vi "Write ready to log boolean.vi"(8 "error in (no error)":errorcluster, 10 "Ready to Log":bool, 11 "Abstract Display in":refnum<class "Abstract Display.lvclass">) -> (0 "error out":errorcluster, 3 "Abstract Display out":refnum<class "Abstract Display.lvclass">)   [LabVIEW 2014, in "Display Panel.lvlib" / "Abstract Display.lvclass"]
uses:
  Abstract Display.lvclass
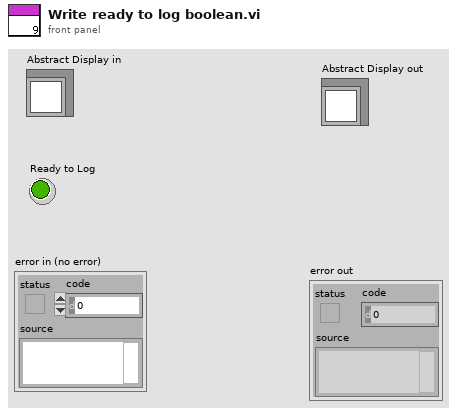
[diagram p1: front panel]
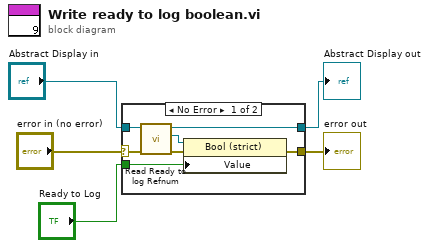
[diagram p0: block diagram]
diagram:
  n1 = case shown="No Error" "error in (no error)" {
    selector: "error in (no error)" -> [w7 w13]
    tunnel: [w12 w13] -> w4
    tunnel: [w10 w14] -> w2
    tunnel: "Abstract Display in" -> [w11 w14]
    tunnel: "Ready to Log" -> [w8 _]
    frame No Error {
      n2 = call-dynamic "Read Ready to log Refnum.vi"("error in (no error)"=w7, "Abstract Display in"=w11) -> ("error out"=w6:errorcluster, "Ready to log Refnum"=w9:refnum<vi>, "Abstract Display out"=w10:refnum<class "Abstract Display.lvclass">)  [unwired: 7 in]
      n3 = property class="Bool (strict)"(reference=w9, error in=w6, "Value"=w8) -> (error out=w12:errorcluster)  [unwired: 1 out]
    }
    frame Error {
    }
  }
  "error out" <- w4
  "Abstract Display out" <- w2
